vi "Camera SelectionToggle Example.vi"() -> ()   [LabVIEW 2017]
uses:
  Global State Variables.vi
panel:
  in  "Boolean 4":bool
  out "Boolean 3":bool
  out "Boolean 2":bool
  in  "Boolean":bool
  out "Camera Selected":enum16{"Peg Camera", "Rope Camera"}(ring)
  in  "Button Ignore Timer":dbl
  in  "stop":bool
  in  "State Selector Methods":enum32{"using one button", "using two buttons"}(tab)
  in  "single buton selector":bool
  in  "right button\nselector":bool
  in  "left button \nselector":bool
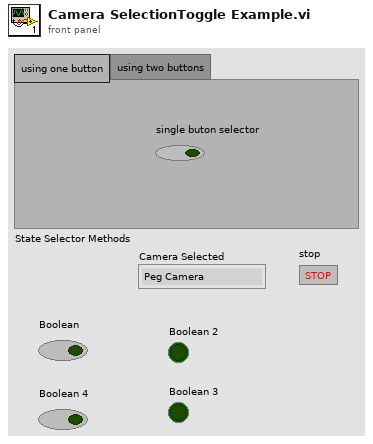
[diagram p1: front panel]
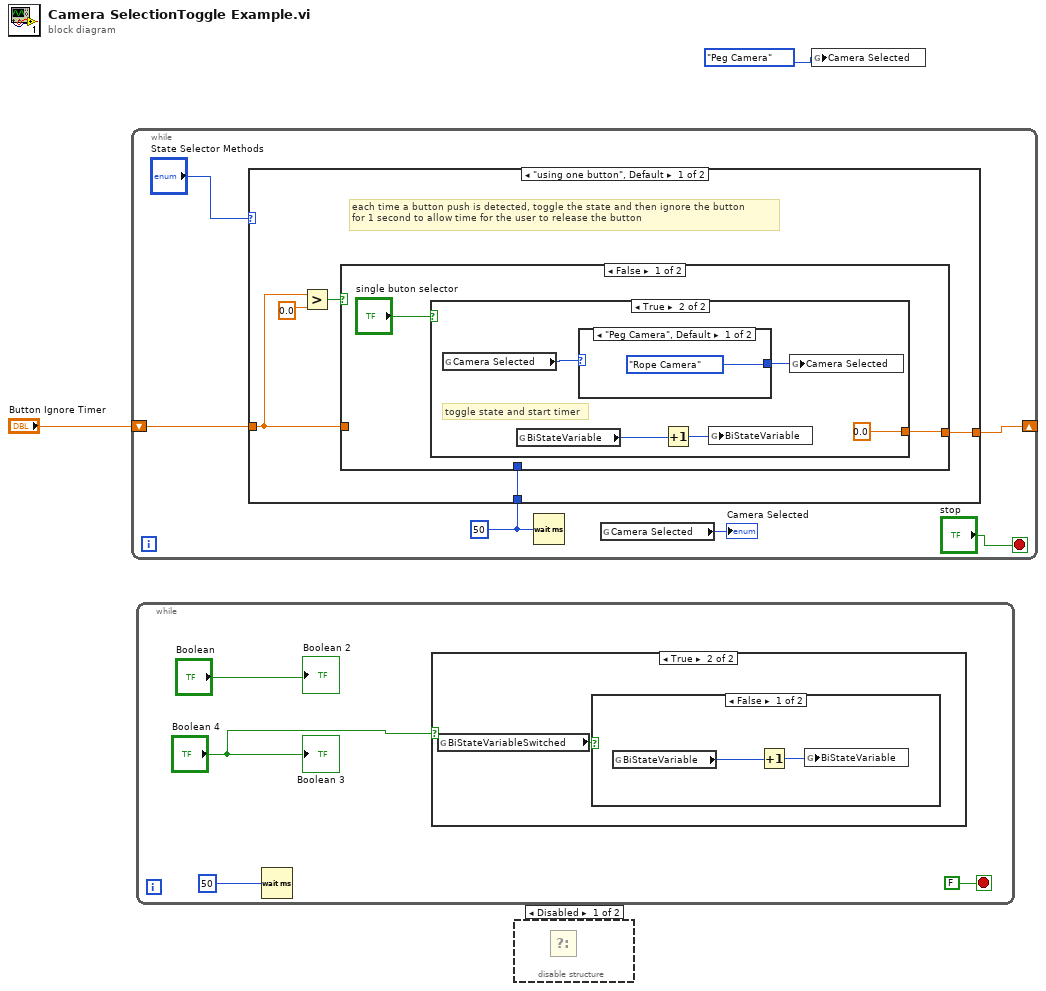
[diagram p0: block diagram]
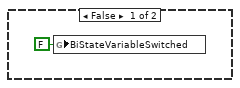
[diagram p3: hidden frame]
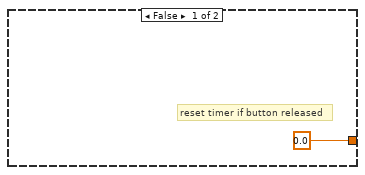
[diagram p5: hidden frame]
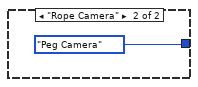
[diagram p6: hidden frame]
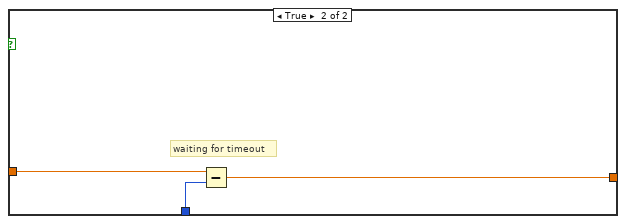
[diagram p7: hidden frame]
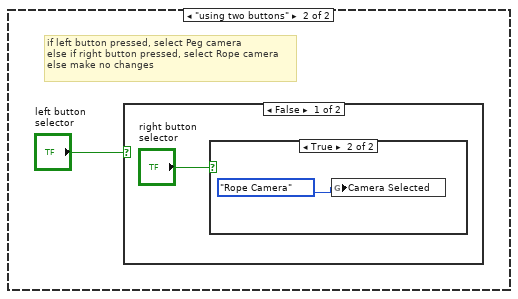
[diagram p8: hidden frame]
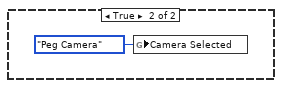
[diagram p10: hidden frame]
diagram:
  n1 = while {
    shift-right: [w4] -> _
    shift-left: "Button Ignore Timer" -> [w6]
    stop <- "stop" stop-if-true
    w5 = u32 50 ("milliseconds to wait")
    n2 = case shown="\"using one button\", Default" "State Selector Methods" {
      tunnel: w6 -> [w11 _]
      tunnel: w5 -> [w10 _]
      tunnel: [w9 _] -> w4
      frame "using one button", Default {
        # "each time a button push is detected, toggle the state and then ignore the button \nfor 1 second to allow time for the user to release the button"
        n3 = Greater?(x=w11, y=0.0) -> (0:w13:bool)
        n4 = case shown="False" w13 {
          tunnel: w11 -> [_ w25]
          tunnel: w10 -> [_ w26]
          tunnel: [w14 w24] -> w9
          frame False {
            n5 = case shown="True" "single buton selector" {
              tunnel: [0.0 ("Button Ignore Timer") 0.0] -> w14
              frame False {
                # "reset timer if button released"
              }
              frame True {
                # "toggle state and start timer"
                n6 = global read "Global State Variables.vi" "Camera Selected"() -> (w21:enum16{"Peg Camera", "Rope Camera"})
                n7 = global read "Global State Variables.vi" "BiStateVariable"() -> (w18:enum16{"State1", "State2"})
                n8 = case shown="\"Peg Camera\", Default" w21 {
                  tunnel: [enum16{"Peg Camera", "Rope Camera"}."Rope Camera" ("Camera Selected") enum16{"Peg Camera", "Rope Camera"}."Peg Camera" ("Camera Selected")] -> w20
                  frame "Peg Camera", Default {
                  }
                  frame "Rope Camera" {
                  }
                }
                n9 = Increment(x=w18) -> (x+1=w17:enum16{"State1", "State2"})
                n10 = global write "Global State Variables.vi" "BiStateVariable"(w17) -> ()
                n11 = global write "Global State Variables.vi" "Camera Selected"(w20) -> ()
              }
            }
          }
          frame True {
            # "waiting for timeout"
            n12 = Subtract(x=w25, y=w26) -> (x-y=w24:dbl)
          }
        }
      }
      frame "using two buttons" {
        # "if left button pressed, select Peg camera\nelse if right button pressed, select Rope camera\nelse make no changes"
        n13 = case shown="False" "left button \nselector" {
          frame False {
            n14 = case shown="True" "right button\nselector" {
              frame False {
              }
              frame True {
                n15 = global write "Global State Variables.vi" "Camera Selected"(enum16{"Peg Camera", "Rope Camera"}."Rope Camera" ("Camera Selected")) -> ()
              }
            }
          }
          frame True {
            n16 = global write "Global State Variables.vi" "Camera Selected"(enum16{"Peg Camera", "Rope Camera"}."Peg Camera" ("Camera Selected")) -> ()
          }
        }
      }
    }
    n17 = Wait (ms)(milliseconds to wait=w5) -> ()  [unwired: 1 out]
    n18 = global read "Global State Variables.vi" "Camera Selected"() -> (→"Camera Selected":enum16{"Peg Camera", "Rope Camera"})
  }
  n19 = while {
    stop <- FALSE stop-if-true
    n20 = Wait (ms)(milliseconds to wait=u32 50) -> ()  [unwired: 1 out]
    n21 = case shown="True" "Boolean 4" {
      frame False {
        n22 = global write "Global State Variables.vi" "BiStateVariableSwitched"(FALSE ("BiStateVariableToggle")) -> ()
      }
      frame True {
        n23 = global read "Global State Variables.vi" "BiStateVariableSwitched"() -> (w36:bool)
        n24 = case shown="False" w36 {
          frame False {
            n25 = global read "Global State Variables.vi" "BiStateVariable"() -> (w38:enum16{"State1", "State2"})
            n26 = Increment(x=w38) -> (x+1=w37:enum16{"State1", "State2"})
            n27 = global write "Global State Variables.vi" "BiStateVariable"(w37) -> ()
          }
          frame True {
          }
        }
      }
    }
    "Boolean 2" <- "Boolean"
    "Boolean 3" <- "Boolean 4"
  }
  n28 = disable-structure shown="Disabled" {
    frame Disabled {
      n29 = Select() -> ()  [unwired: 3 in, 1 out]
    }
    frame Enabled {
    }
  }
  n30 = global write "Global State Variables.vi" "Camera Selected"(enum16{"Peg Camera", "Rope Camera"}."Peg Camera" ("Camera Selected")) -> ()
